vi "DAQ@Display2User__Parameter.vi"(1 "ParamterIn":string) -> (0 "ParamterOut":string)   [LabVIEW 2020]
panel:
  in  "UserControlName":string(combo)
  in  "WaveFormName":string(combo)
  in  "Confirm":bool
  # "DAQ@Display2User $WaveFormName,$UserPanleControlName"
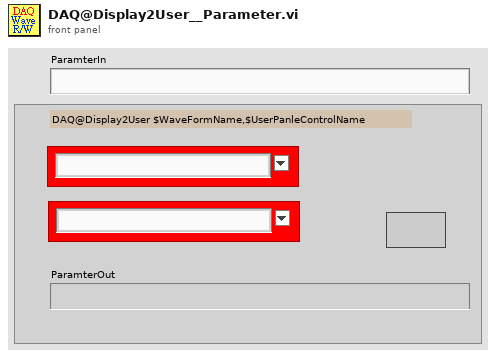
[diagram p1: front panel]
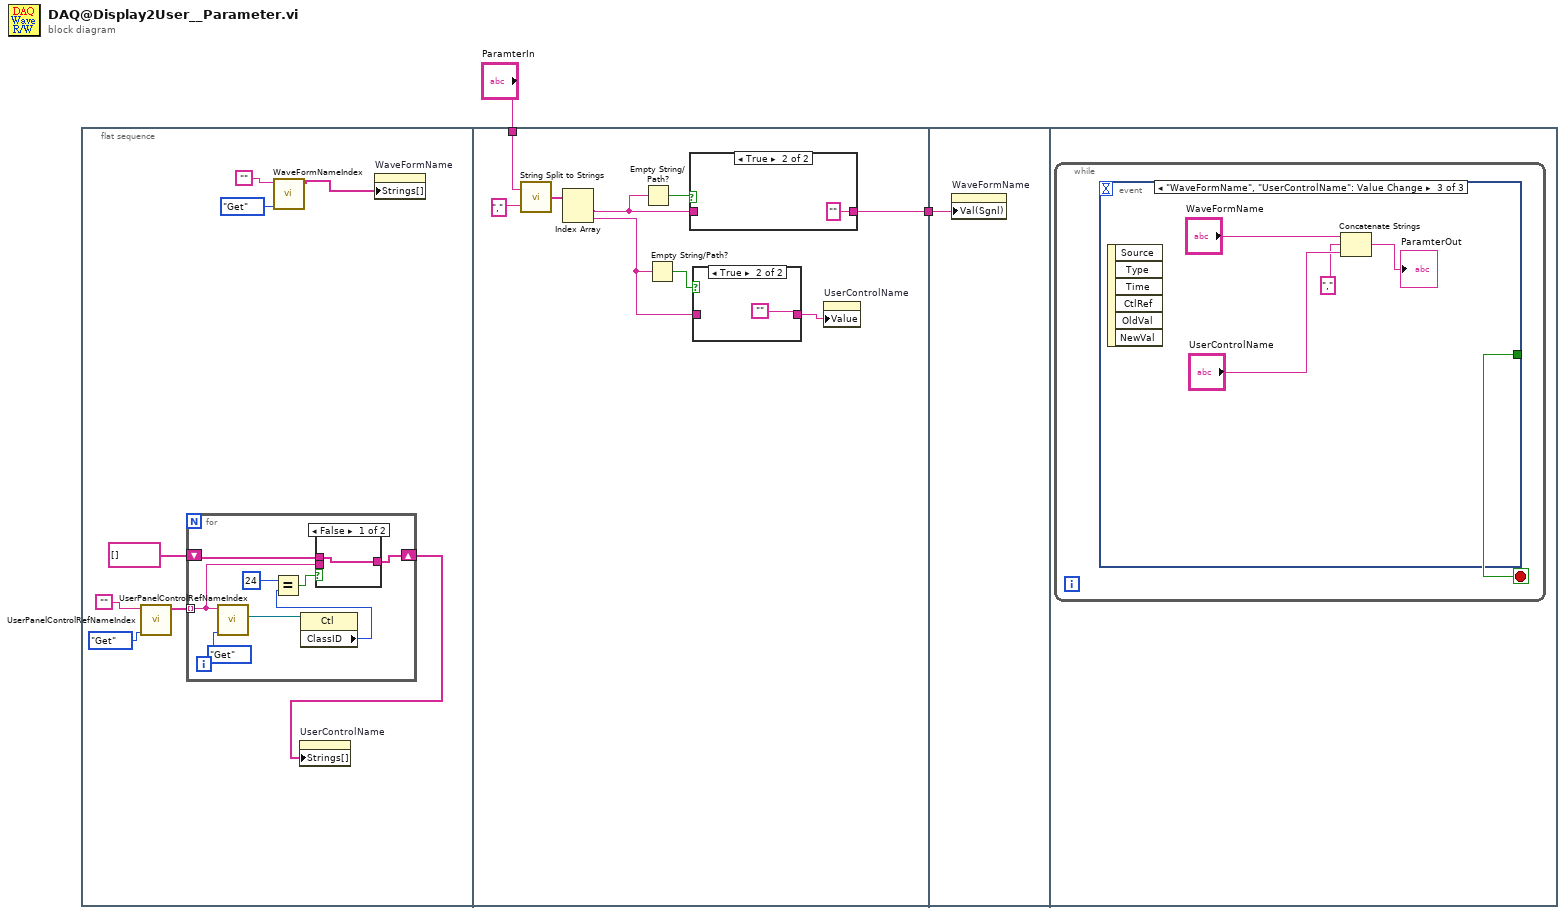
[diagram p0: block diagram]
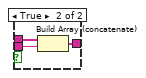
[diagram p2: hidden frame]
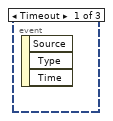
[diagram p5: hidden frame]
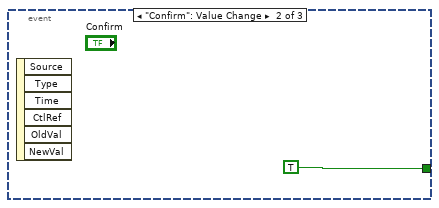
[diagram p6: hidden frame]
diagram:
  n1 = flat-sequence {
    tunnel: "ParamterIn" -> [w28]
    tunnel: [w23] -> w1
    tunnel: w1 -> [w36]
    frame #0 {
      n2 = call "UserPanelControlRefNameIndex.vi"("OP"=enum16{"Get", "Update", "Init"}."Get", "ControlName"="") -> ("ControlNameS"=w7:string[])  [unwired: 6 in, 3 out]
      n3 = for {
        tunnel: w7 -> [w13] mode=indexing
        shift-right: [w12] -> w3
        shift-left: string[] [] ("Strings []") -> [w14]
        n4 = call "UserPanelControlRefNameIndex.vi"("OP"=enum16{"Get", "Update", "Init"}."Get", "ControlName"=w13) -> ("ControlRefOut"=w17:refnum<vi>)  [unwired: 6 in, 3 out]
        n5 = property class="Ctl"(reference=w17) -> ("ClassID"=w16:u32)  [unwired: 1 in, 2 out]
        n6 = Equal?(x=u32 24, y=w16) -> (x = y?=w15:bool)
        n7 = case shown="False" w15 {
          tunnel: w14 -> [w19 w22]
          tunnel: w13 -> [_ w21]
          tunnel: [w19 w20] -> w12
          frame False {
          }
          frame True {
            n8 = Build Array (concatenate)(w22, w21) -> (w20:string[])
          }
        }
      }
      n9 = call "WaveFormNameIndex.vi"("OP"=enum16{"Get", "Update", "Init", "GetSPS"}."Get", "WaveFormName"="") -> ("WaveFormNameList"=w8:string[])  [unwired: 6 in, 3 out]
      n10 = property on="UserControlName" class="CmbBox"("Strings[]"=w3) -> ()  [unwired: 2 in, 2 out]
      n11 = property on="WaveFormName" class="CmbBox"("Strings[]"=w8) -> ()  [unwired: 2 in, 2 out]
    }
    frame #1 {
      n12 = call "String Split to Strings.vi"("search string/char (-)"=",", "String"=w28) -> ("Array"=w30:string[])
      n13 = Index Array(array=w30) -> (element #1=w27:string, element #2=w24:string)  [unwired: 2 in]
      n14 = Empty String/Path?(string/path=w27) -> (empty?=w31:bool)
      n15 = Empty String/Path?(string/path=w24) -> (empty?=w26:bool)
      n16 = case shown="True" w31 {
        tunnel: w27 -> [w34 _]
        tunnel: [w34 ""] -> w23
        frame False {
        }
        frame True {
        }
      }
      n17 = case shown="True" w26 {
        tunnel: [w32 ""] -> w25
        tunnel: w24 -> [w32 _]
        frame False {
        }
        frame True {
        }
      }
      n18 = property on="UserControlName" class="CmbBox"("Value"=w25) -> ()  [unwired: 2 in, 2 out]
    }
    frame #2 {
      n19 = property on="WaveFormName" class="CmbBox"("Val(Sgnl)"=w36) -> ()  [unwired: 2 in, 2 out]
    }
    frame #3 {
      n20 = while {
        stop <- w37 stop-if-true
        n21 = event shown="[2] \"WaveFormName\", \"UserControlName\": Value Change" {
          selector: _ -> [_ _ _]
          dyn-events: _ -> [_ _ _]
          timeout: _ -> [_ _ _]
          tunnel: [_ TRUE _] -> w37
          event Timeout {
            n22 = event-data() -> ()  [unwired: 1 in, 3 out]
          }
          event "Confirm": Value Change {
            n23 = event-data() -> ()  [unwired: 1 in, 6 out]
          }
          event "WaveFormName", "UserControlName": Value Change {
            n24 = event-data() -> ()  [unwired: 1 in, 6 out]
            n25 = Concatenate Strings("WaveFormName", ",", "UserControlName") -> (→"ParamterOut":string)
          }
        }
      }
    }
  }
